vi "Run.vi"(8 "error in (no error)":errorcluster, 11 "FormulaLV App in":refnum<class "FormulaG App.lvclass">) -> (0 "error out":errorcluster, 3 "FormulaLV App out":refnum<class "FormulaG App.lvclass">)   [LabVIEW 2024, in "FormulaG.lvlib" / "FormulaG App.lvclass"]
uses:
  FormulaG App.lvclass
  FormulaG App.lvclass/FormulaG App.ctl
  <vilib>/IlluminatedG/IG GodotServer/GodotLV/GodotServer/GodotServer.lvclass
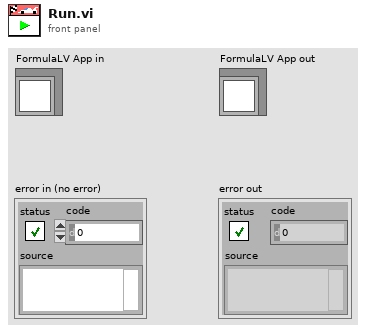
[diagram p1: front panel]
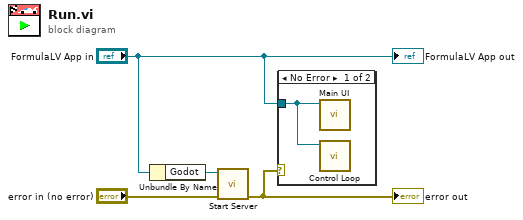
[diagram p0: block diagram]
diagram:
  n1 = Unbundle By Name("FormulaLV App in") -> ("Godot"=w3:refnum<class "GodotServer.lvclass">)
  n2 = call <vilib>:"Start Server.vi"("error in (no error)"="error in (no error)", "GodotServer in"=w3) -> ("error out"=w1:errorcluster)  [unwired: 8 in, 1 out]
  "error out" <- w1
  n3 = case shown="No Error" w1 {
    tunnel: "FormulaLV App in" -> [w5 _]
    frame No Error {
      n4 = call "Main UI.vi"("FormulaLV App in"=w5) -> ()  [unwired: 11 in]
      n5 = call "Control Loop.vi"("FormulaG App in"=w5) -> ()  [unwired: 10 in, 1 out]
    }
    frame Error {
    }
  }
  "FormulaLV App out" <- "FormulaLV App in"
